vi "Find Entity by Type.vi"(7 "Entity Type":refnum<class "Entity.lvclass">, 8 "error in (no error)":errorcluster, 10 "Type":refnum<class "Type.lvclass">, 11 "Entity Manager in":refnum<class "Entity Manager.lvclass">) -> (0 "error out":errorcluster, 2 "Entity":refnum<class "Entity.lvclass">, 3 "Entity Manager out":refnum<class "Entity Manager.lvclass">)   [LabVIEW 2020, in "Conditu2.lvlib" / "Entity Manager.lvclass"]
uses:
  Entity Manager.lvclass
  Entity/Entity.lvclass
  Columns/Type/Type.lvclass
  Entity Manager.lvclass/Entity Manager.ctl
  Entity/Set From Result Row.vi
  Database Platform/Database Platform.lvclass
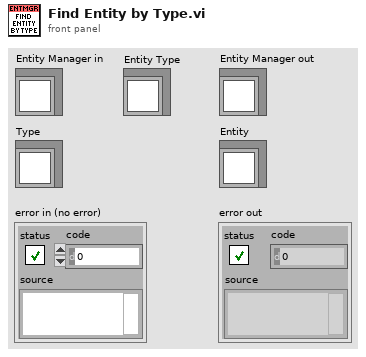
[diagram p1: front panel]
types:
  T1 = typedef "Conditu2.lvlib/Entity Manager.lvclass/Known Entity.ctl" = cluster{"Entity":refnum<class "Entity.lvclass">, "Types":refnum<class "Type.lvclass">[], "Type Name Map":map{string, i32}}
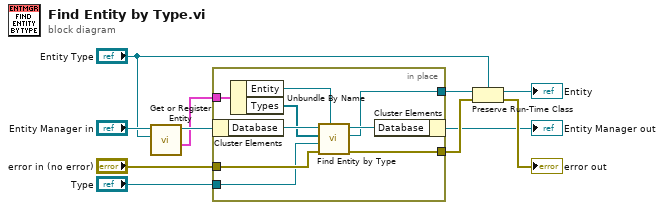
[diagram p0: block diagram]
diagram:
  n1 = call "Get or Register Entity.vi"("Entity"="Entity Type", "Entity Manager in"="Entity Manager in") -> ("Entity Info"=w4:T1, "Entity Manager out"=w5:refnum<class "Entity Manager.lvclass">)  [unwired: 8 in]
  n2 = in-place {
    in-place-border: "Type" -> [w16]
    in-place-border: "error in (no error)" -> [w19]
    in-place-border: [w17] -> w11
    in-place-border: w4 -> [w15]
    in-place-border: [w12] -> w3
    n3 = in-place-cluster #1(w5) -> ("Database"=w20:refnum<class "Database Platform.lvclass">)
    n4 = Unbundle By Name(w15) -> ("Entity"=w14:refnum<class "Entity.lvclass">, "Types"=w13:refnum<class "Type.lvclass">[])
    n5 = call "Find Entity by Type.vi"("Entity Type"=w14, "error in (no error)"=w19, "Column Criteria"=w16, "Types"=w13, "Database in"=w20) -> ("error out"=w17:errorcluster, "Entity"=w12:refnum<class "Entity.lvclass">, "Database out"=w18:refnum<class "Database Platform.lvclass">)  [unwired: 4 in]
    n6 = in-place-cluster #1("Database"=w18) -> (→"Entity Manager out":refnum<class "Entity Manager.lvclass">)
  }
  n7 = Preserve Run-Time Class(object in=w3, error in=w11, 2:"Entity Type") -> (object out=→"Entity":refnum<class "Entity.lvclass">, error out=→"error out":errorcluster)
